vi "차선 클러스터 분리.vi"(1 "배열":cluster{"X":sgl, "Y":sgl}[](array[cluster])) -> (0 "R, Theta":dbl[](array[numeric]))   [LabVIEW 2016]
uses:
  <vilib>/ptbypt/NI_PtbyPt.lvlib
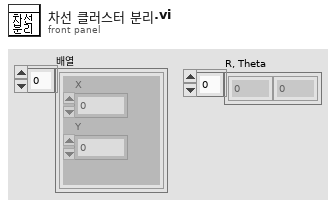
[diagram p1: front panel]
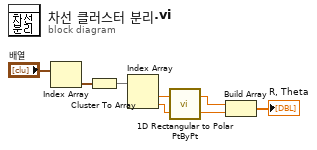
[diagram p0: block diagram]
diagram:
  n1 = Index Array(array="배열") -> (element=w8:cluster{"X":sgl, "Y":sgl})  [unwired: 1 in]
  n2 = Cluster To Array(cluster=w8) -> (array=w7:sgl[])
  n3 = Index Array(array=w7) -> (element #1=w6:sgl, element #2=w5:sgl)  [unwired: 2 in]
  n4 = call <vilib>:"1D Rectangular to Polar PtByPt.vi"("y"=w5, "x"=w6) -> ("phase"=w2:dbl, "magnitude"=w3:dbl)
  n5 = Build Array(w3, w2) -> (→"R, Theta":dbl[])
